vi "Init PWM Waveform.vi"(8 "error in":errorcluster, 9 "Duty Cycle":dbl=10.0 format="%0.2p %", 10 "Frequency":dbl=10.0 format="%0.2p Hz", 11 "DO DAQmx Fixed Freq PWM CFG in":refnum<class "DO DAQmx Fixed Freq PWM CFG.lvclass">) -> (0 "error out":errorcluster, 2 "PWM Waveform":digitalwaveform(waveform), 3 "DO DAQmx Fixed Freq PWM CFG out":refnum<class "DO DAQmx Fixed Freq PWM CFG.lvclass">)   [LabVIEW 2023, in "DO DAQmx Fixed Freq PWM CFG.lvclass"]
uses:
  DO DAQmx Fixed Freq PWM CFG.lvclass
  Configuration/Configuration JSON/Configuration JSON Base/CFG JSON.lvclass/CFG JSON.ctl
  DO DAQmx Fixed Freq PWM CFG.lvclass/DO DAQmx Fixed Freq PWM CFG.ctl
  501ba0a0-c2c9-46ab-a0a9-86892fbf8d4b.vi
  <vilib>/JDP Science/JSONtext/Find Item.vi
  <vilib>/JDP Science/JSONtext/Next JSON Value.vi
  <vilib>/JDP Science/JSONtext/String Subset.vi
  <vilib>/JDP Science/JSONtext/Parsing/Advance past next JSON Value (inlined COPY).vi
  <vilib>/JDP Science/JSONtext/Parsing/Advance past whitespace.vi
  <vilib>/JDP Science/JSONtext/Parsing/Advance past String.vi
  <vilib>/JDP Science/JSONtext/Parsing/Advance past Number.vi
  <vilib>/JDP Science/JSONtext/Parsing/Advance past Line Ending.vi
  <vilib>/JDP Science/JSONtext/Parsing/Parse Full Path or Item Name.vi
  <vilib>/JDP Science/JSONtext/Parsing/Advance past Array.vi
  <vilib>/JDP Science/JSONtext/Parsing/Advance past Object.vi
  <vilib>/JDP Science/JSONtext/support/Error Cluster From Code.vi
  <vilib>/JDP Science/JSONtext/Offset/Find Item Locations by Path.vi
  <vilib>/JDP Science/JSONtext/JSON text to Variant.vi
  <vilib>/Utility/error.llb/Error Cluster From Error Code.vi
  <vilib>/JDP Science/JSONtext/LVClass Serializer/JSONtext LVClass Serializer.lvclass
  <vilib>/ErrorRing/Error Ring.xnode
  Configuration/Configuration JSON/Configuration JSON Base/CFG JSON.lvclass
  D:/git/HAL/HAL GOOP4/DAQmx/DAQmx Base CFG/DAQmx Base CFG.lvclass
  D:/git/HAL/HAL GOOP4/CFG Target/CFG Target.lvclass
  D:/git/HAL/HAL GOOP4/Configuration/Configuration Semaphore/CFG Semaphore.lvclass
  D:/git/HAL/HAL GOOP4/Configuration/Configuration JSON/Configuration JSON Base/CFG JSON.lvclass
  D:/git/HAL/HAL GOOP4/Interfaces/IConfigure/IConfigure.lvclass
  D:/git/HAL/HAL GOOP4/DIO/DO DAQmx Fixed Freq PWM CFG/DO DAQmx Fixed Freq PWM CFG.lvclass
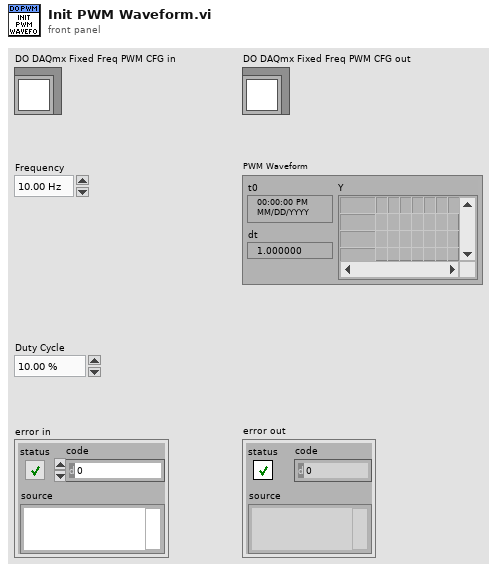
[diagram p1: front panel]
types:
  T1 = cluster{"Samples per Channel":i32, "Samplerate":dbl}
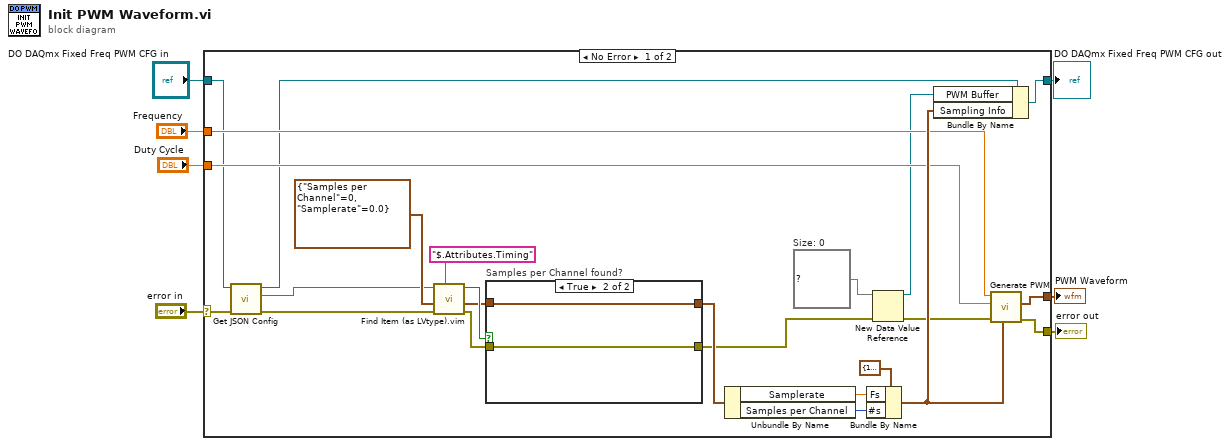
[diagram p0: block diagram]
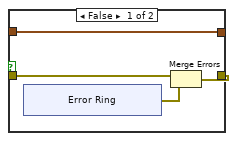
[diagram p2: hidden frame]
diagram:
  n1 = case shown="No Error" "error in" {
    selector: "error in" -> [w12 w43]
    tunnel: [w25 _] -> w7
    tunnel: [w24 w43] -> w6
    tunnel: [w20 w44] -> w5
    tunnel: "Frequency" -> [w18 _]
    tunnel: "Duty Cycle" -> [w17 _]
    tunnel: "DO DAQmx Fixed Freq PWM CFG in" -> [w15 w44]
    frame No Error {
      w11 = map{string, digitalwaveform} {}  # Size: 0
      n2 = call "Get JSON Config.vi"("error in (no error)"=w12, "CFG Base in"=w15) -> ("error out"=w16:errorcluster, "<JSON>Config>"=w13:string, "CFG Base out"=w14:refnum<class "DO DAQmx Fixed Freq PWM CFG.lvclass">)  [unwired: 7 in]
      n3 = call "Find Item (as LVtype).vim"("$Path or Item Name"="$.Attributes.Timing", "error in (no error)"=w16, "Data Type and Default Value"=T1 {"Samples per Channel"=0, "Samplerate"=0.0}, "JSON"=w13) -> ("error out"=w30:errorcluster, "Data"=w29:T1, "Found"=w31:bool)  [unwired: 4 in, 1 out]
      n4 = case "Samples per Channel found?" shown="True" w31 {
        tunnel: w30 -> [w34 w42]
        tunnel: [w33 w42] -> w10
        tunnel: w29 -> [w32 w41]
        tunnel: [w32 w41] -> w26
        frame False {
          n5 = xnode "Error Ring"() -> ("error out"=w35:errorcluster)
          n6 = Merge Errors(w34, w35) -> (w33:errorcluster)
        }
        frame True {
        }
      }
      n7 = Unbundle By Name(w26) -> ("Samplerate"=w22:dbl, "Samples per Channel"=w21:i32)
      n8 = Bundle By Name(cluster=cluster{"Fs":dbl, "#s":dbl} {"Fs"=1000.0, "#s"=1000.0} ("sampling info"), "Fs"=w22, "#s"=w21) -> (w19:cluster{"Fs":dbl, "#s":dbl})
      n9 = New Data Value Reference(data value=w11, error in=w10) -> (data value reference=w8:refnum<data-value>, error out=w9:errorcluster)
      n10 = Bundle By Name(cluster=w14, "PWM Buffer"=w8, "Sampling Info"=w19) -> (w20:refnum<class "DO DAQmx Fixed Freq PWM CFG.lvclass">)
      n11 = call "Generate PWM.vi"("sampling info"=w19, "error in"=w9, "duty cycle"=w17, "frequency"=w18) -> ("error out"=w24:errorcluster, "digital waveform"=w25:digitalwaveform)  [unwired: 6 in]
    }
    frame Error {
    }
  }
  "PWM Waveform" <- w7
  "error out" <- w6
  "DO DAQmx Fixed Freq PWM CFG out" <- w5
